vi "CTRE_Phoenix_CANcoder_ClearStickyFaults.vi"(6 "timoutMs":i32, 8 "error in":errorcluster, 11 "CTRE_CANcoder_DeviceRef":T1) -> (0 "error out":errorcluster, 3 "CTRE_CANcoder_DeviceRef":T1)   [LabVIEW 2019]
doc: "Clears the sticky faults in the CANcoder."
uses:
  <vilib>/Rock Robotics/WPI/ThirdParty/Phoenix-LabVIEW/CANCoder/Controls/CTRE_Phoenix_CANcoder_DeviceRef.ctl
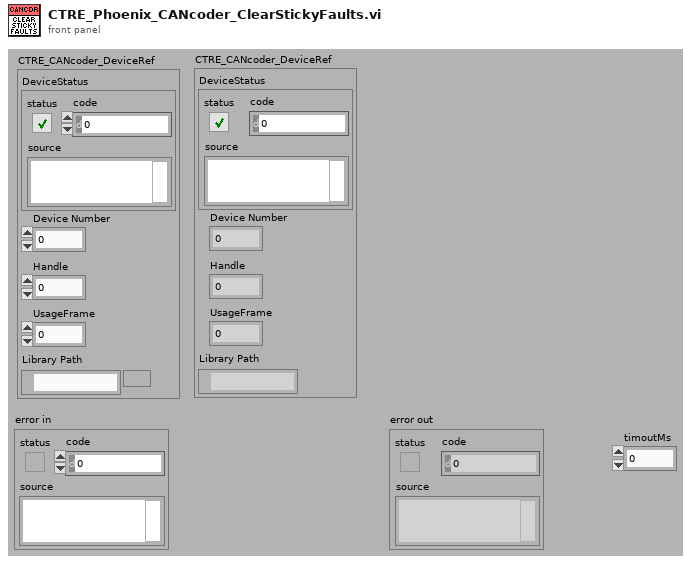
[diagram p1: front panel]
types:
  T1 = typedef "CTRE_Phoenix_CANcoder_DeviceRef.ctl" = cluster{"DeviceStatus":errorcluster, "Device Number":u8, "Handle":u64, "UsageFrame":u32, "Library Path":path}
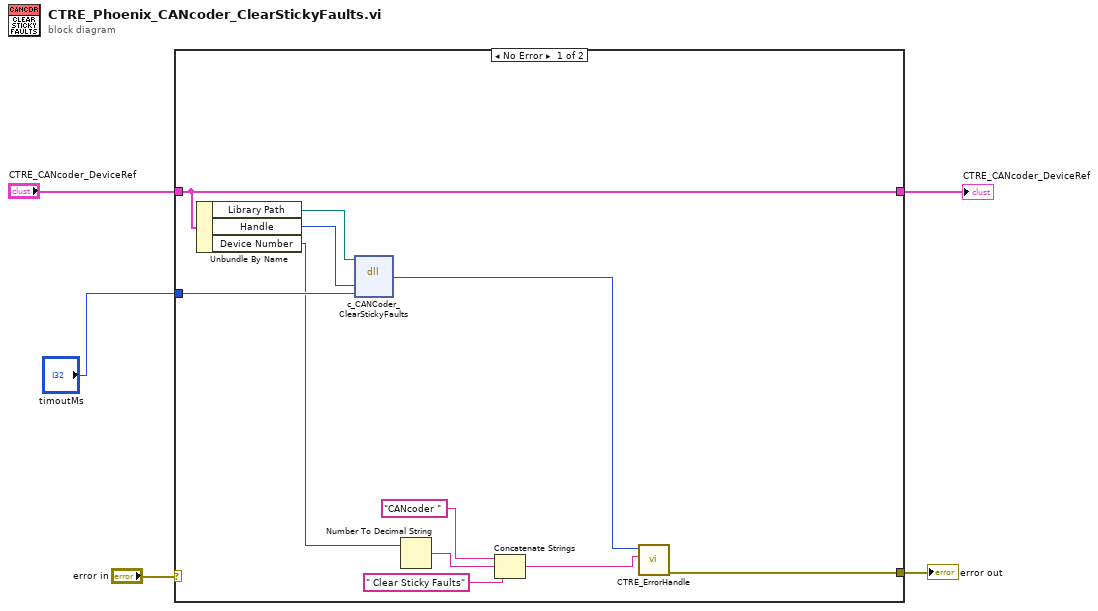
[diagram p0: block diagram]
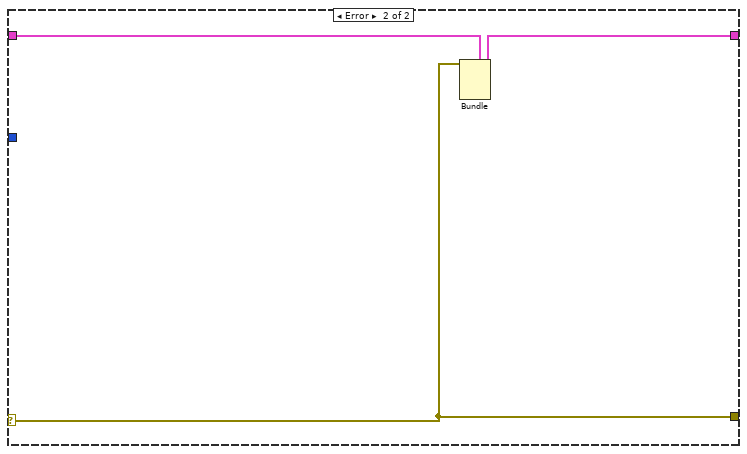
[diagram p2: hidden frame]
diagram:
  n1 = case shown="No Error" "error in" {
    selector: "error in" -> [_ w18]
    tunnel: "CTRE_CANcoder_DeviceRef" -> [w13 w19]
    tunnel: [w16 w18] -> w5
    tunnel: [w13 w17] -> w2
    tunnel: "timoutMs" -> [w14 _]
    frame No Error {
      n2 = Unbundle By Name(w13) -> ("Library Path"=w11:path, "Handle"=w12:u64, "Device Number"=w6:u8)
      n3 = dll-call lib="?" fn="c_CANCoder_ClearStickyFaults"(path in=w11, "handle"=w12, "timoutMs"=w14) -> ("ErrorCode"=w15:i32)  [unwired: 4 in, 2 out]
      n4 = Number To Decimal String(number=w6) -> (decimal integer string=w10:string)  [unwired: 1 in]
      n5 = Concatenate Strings("CANcoder " ("string"), w10, " Clear Sticky Faults" ("string")) -> (w8:string)
      n6 = call <vilib>:"CTRE_ErrorHandle.vi"("origin"=w8, "code"=w15) -> ("error out"=w16:errorcluster)  [unwired: 9 in]
    }
    frame Error {
      n7 = Bundle(cluster=w19, "DeviceStatus"=w18) -> (w17:T1)  [unwired: 4 in]
    }
  }
  "error out" <- w5
  "CTRE_CANcoder_DeviceRef" <- w2
